vi "InsideObstruction.vi"(8 "error in (no error)":errorcluster, 10 "point":cluster{"X":dbl, "Y":dbl}, 11 "Polygon in":refnum<class "Polygon.lvclass">) -> (0 "error out":errorcluster, 2 "inside":bool, 3 "Polygon out":refnum<class "Polygon.lvclass">)   [LabVIEW 2014, in "Polygon.lvclass"]
uses:
  <userlib>/AdvancedDataStructures/ClassBased/Applications/Occupancy/Polygon/Polygon.lvclass
  <userlib>/AdvancedDataStructures/ClassBased/Applications/Occupancy/Polygon/Polygon.lvclass/Polygon.ctl
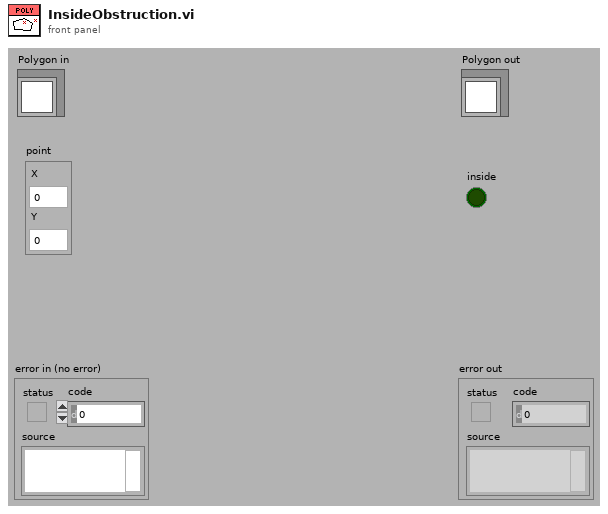
[diagram p1: front panel]
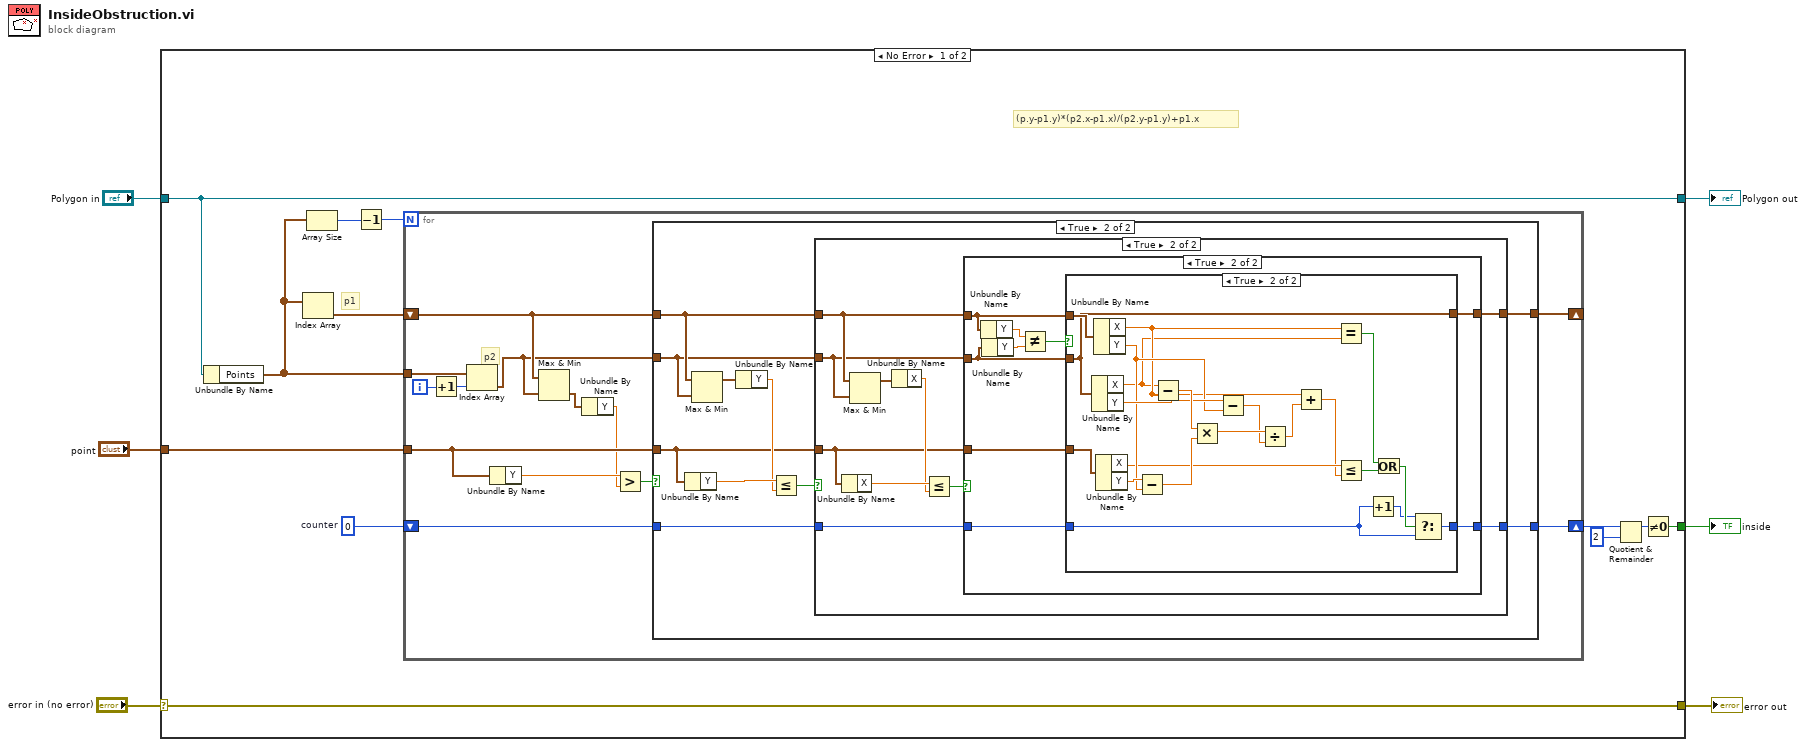
[diagram p0: block diagram]
diagram:
  n1 = case shown="No Error" "error in (no error)" {
    selector: "error in (no error)" -> [w18 w91]
    tunnel: [w18 w91] -> w3
    tunnel: [w17 w90] -> w1
    tunnel: "Polygon in" -> [w17 w90]
    tunnel: "point" -> [w7 _]
    tunnel: [w11 _] -> w2
    frame No Error {
      w15 = 0  # counter
      # "(p.y-p1.y)*(p2.x-p1.x)/(p2.y-p1.y)+p1.x"
      # "p1"
      n2 = Unbundle By Name(w17) -> ("Points"=w8:cluster{"X":dbl, "Y":dbl}[])
      n3 = Index Array(array=w8) -> (element=w16:cluster{"X":dbl, "Y":dbl})  [unwired: 1 in]
      n4 = Array Size(array=w8) -> (size(s)=w9:i32)
      n5 = Decrement(x=w9) -> (x-1=w10:i32)
      n6 = for {
        N: w10 -> [_]
        shift-right: [w19] -> _
        shift-left: w16 -> [w26]
        tunnel: w7 -> [w22]
        tunnel: w8 -> [w29]
        shift-right: [w27] -> w14
        shift-left: w15 -> [w28]
        i -> [w31]
        # "p2"
        n7 = Increment(x=w31) -> (x+1=w30:i32)
        n8 = Index Array(array=w29, index=w30) -> (element=w25:cluster{"X":dbl, "Y":dbl})
        n9 = Unbundle By Name(w22) -> ("Y"=w24:dbl)
        n10 = Max & Min(x=w26, y=w25) -> (min(x,y)=w21:cluster{"X":dbl, "Y":dbl})  [unwired: 1 out]
        n11 = Unbundle By Name(w21) -> ("Y"=w20:dbl)
        n12 = Greater?(x=w24, y=w20) -> (0:w23:bool)
        n13 = case shown="True" w23 {
          tunnel: w26 -> [_ w41]
          tunnel: w25 -> [w33 w40]
          tunnel: w28 -> [w32 w43]
          tunnel: [w32 w42] -> w27
          tunnel: w22 -> [_ w35]
          tunnel: [w33 w34] -> w19
          frame False {
          }
          frame True {
            n14 = Unbundle By Name(w35) -> ("Y"=w38:dbl)
            n15 = Max & Min(x=w41, y=w40) -> (max(x,y)=w39:cluster{"X":dbl, "Y":dbl})  [unwired: 1 out]
            n16 = Unbundle By Name(w39) -> ("Y"=w37:dbl)
            n17 = Less Or Equal?(x=w38, y=w37) -> (x <= y?=w36:bool)
            n18 = case shown="True" w36 {
              tunnel: w41 -> [_ w52]
              tunnel: w40 -> [w45 w51]
              tunnel: w43 -> [w44 w55]
              tunnel: [w44 w54] -> w42
              tunnel: w35 -> [_ w47]
              tunnel: [w45 w46] -> w34
              frame False {
              }
              frame True {
                n19 = Unbundle By Name(w47) -> ("X"=w53:dbl)
                n20 = Max & Min(x=w52, y=w51) -> (max(x,y)=w50:cluster{"X":dbl, "Y":dbl})  [unwired: 1 out]
                n21 = Unbundle By Name(w50) -> ("X"=w49:dbl)
                n22 = Less Or Equal?(x=w53, y=w49) -> (x <= y?=w48:bool)
                n23 = case shown="True" w48 {
                  tunnel: w52 -> [_ w59]
                  tunnel: w51 -> [w57 w60]
                  tunnel: w55 -> [w56 w63]
                  tunnel: [w56 w62] -> w54
                  tunnel: w47 -> [_ w61]
                  tunnel: [w57 w58] -> w46
                  frame False {
                  }
                  frame True {
                    n24 = Unbundle By Name(w59) -> ("Y"=w65:dbl)
                    n25 = Unbundle By Name(w60) -> ("Y"=w66:dbl)
                    n26 = Not Equal?(x=w65, y=w66) -> (x != y?=w64:bool)
                    n27 = case shown="True" w64 {
                      tunnel: w63 -> [w67 w70]
                      tunnel: [w67 w69] -> w62
                      tunnel: w61 -> [_ w89]
                      tunnel: w60 -> [w68 w73]
                      tunnel: w59 -> [_ w88]
                      tunnel: [w68 w73] -> w58
                      frame False {
                      }
                      frame True {
                        n28 = Unbundle By Name(w73) -> ("X"=w78:dbl, "Y"=w84:dbl)
                        n29 = Unbundle By Name(w88) -> ("X"=w79:dbl, "Y"=w83:dbl)
                        n30 = Unbundle By Name(w89) -> ("X"=w77:dbl, "Y"=w87:dbl)
                        n31 = Subtract(x=w87, y=w83) -> (x-y=w86:dbl)
                        n32 = Subtract(x=w78, y=w79) -> (x-y=w85:dbl)
                        n33 = Multiply(x=w85, y=w86) -> (x*y=w82:dbl)
                        n34 = Subtract(x=w84, y=w83) -> (x-y=w81:dbl)
                        n35 = Divide(x=w82, y=w81) -> (x/y=w80:dbl)
                        n36 = Add(x=w79, y=w80) -> (x+y=w76:dbl)
                        n37 = Equal?(x=w79, y=w78) -> (x = y?=w75:bool)
                        n38 = Less Or Equal?(x=w77, y=w76) -> (x <= y?=w74:bool)
                        n39 = Increment(x=w70) -> (x+1=w71:i32)
                        n40 = Or(x=w75, y=w74) -> (x .or. y?=w72:bool)
                        n41 = Select(t=w71, s=w72, f=w70) -> (s? t:f=w69:i32)
                      }
                    }
                  }
                }
              }
            }
          }
        }
      }
      n42 = Quotient & Remainder(x=w14, y=2) -> (x-y*floor(x/y)=w12:i32)  [unwired: 1 out]
      n43 = Not Equal To 0?(x=w12) -> (x != 0?=w11:bool)
    }
    frame Error {
    }
  }
  "error out" <- w3
  "Polygon out" <- w1
  "inside" <- w2
